vi "FTW-CodeGen-GetTerminals.vi"(0 "Prototype VI":refnum<vi>, 11 "error in":errorcluster) -> (4 "Terms":T5(array[cluster]), 6 "Adaptive Input Terminals":T1[](array[typedef]), 15 "error out":errorcluster)   [LabVIEW 2015]
uses:
  FTW-CodeGen-XNodeAdaptiveTerminal.ctl
  FTW-CodeGen-XNodeAdaptiveTerminal-Controller.ctl
  src/reflection/FTW-Reflection-Types.ctl
  FTW-CodeGen-XNodeAdaptiveTerminal-ControllerBehavior.ctl
  FTW-CodeGen-XNodeAdaptiveTerminal-Dependent.ctl
panel:
  # "Inputs"
  # "Outputs"
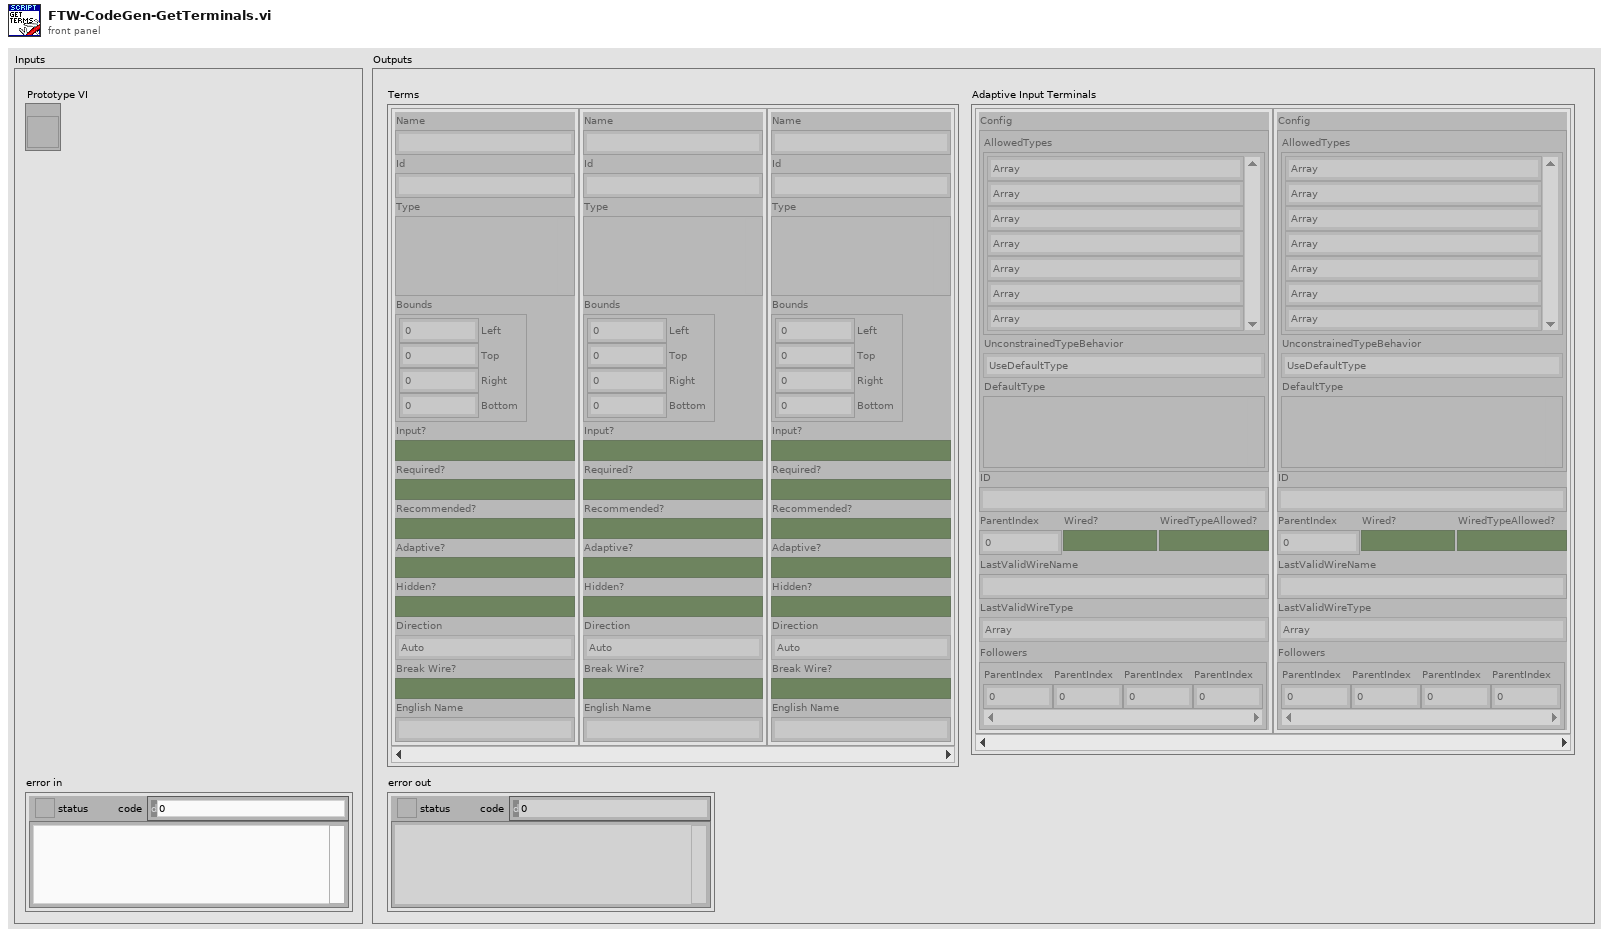
[diagram p1: front panel]
types:
  T1 = typedef "FTW-CodeGen-XNodeAdaptiveTerminal.ctl" = cluster{"Config":T2, "ID":string, "ParentIndex":i32, "Wired?":bool, "WiredTypeAllowed?":bool, "LastValidWireName":string, "LastValidWireType":T3, "Followers":i32[]}
  T2 = typedef "FTW-CodeGen-XNodeAdaptiveTerminal-Controller.ctl" = cluster{"AllowedTypes":T3[], "UnconstrainedTypeBehavior":T4, "DefaultType":variant}
  T3 = typedef "FTW-Reflection-Types.ctl" = enum16{"Unknown", "Void", "Array", "Cluster", "LVObject", "Boolean", "I8", "I16", "I32", "I64", "U8", "U16", "U32", "U64", "SGL", "DBL", "EXT", "CSG", "CDB", "CXT", "FXP", "EnumU8", "EnumU16", "EnumU32", "EnumU64", "SGLwithUnit", "DBLwithUnit", "EXTwithUnit", "CSGwithUnit", "CDBwithUnit", "CXTwithUnit", "String", "Path", "Picture", "Tag", "LVVariant", "Timestamp", "WaveformI8", "WaveformI16", "WaveformI32", "WaveformI64", "WaveformU8", "WaveformU16", "WaveformU32", "WaveformU64", "WaveformSGL", "WaveformDBL", "WaveformEXT", "WaveformCSG", "WaveformCDB", "WaveformCXT", "WaveformDigital", "WaveformUnknownType", "DigitalData", "DynamicData", "ExternalData", "FileByteStream", "TDMStream", "dotNET", "ActiveX", "VIServerReference", "VIReference", "ApplicationInstance", "Menu", "ConnectionDataSocket", "ConnectionVISA", "ConnectionBluetooth", "ConnectionIrDA", "ConnectionTCP", "ConnectionUDP", "ConnectionHTTPClient", "ConnectionFTP", "Occurrence", "Notifier", "Queue", "Rendezvous", "Semaphore", "RTFIFO", "EventPublisher", "EventRegistration", "EventCallback", "DataValueReference", "GenericClass", "GenericClassTag", "GenericClassDeepCopy", "GenericClassFlattened", "GenericClassTagFlattened", "GenericReferenceType", "WindowsRegistry", "OverloadedDatalogRef", "ReferenceUnknownType", "ByteArray", "ConPaneInterface", "FTWObject"}
  T4 = typedef "FTW-CodeGen-XNodeAdaptiveTerminal-ControllerBehavior.ctl" = enum16{"UseDefaultType", "StickyToLastValidType"}
  T5 = cluster{"Name":string, "Id":string, "Type":variant, "Bounds":cluster{"Left":i32, "Top":i32, "Right":i32, "Bottom":i32}, "Input?":bool, "Required?":bool, "Recommended?":bool, "Adaptive?":bool, "Hidden?":bool, "Direction":enum32{"Auto", "Up", "Down", "Left", "Right", "Center"}, "Break Wire?":bool, "English Name":string}[]
  T6 = typedef "FTW-Reflection-ConPaneInterface-Terminal.ctl" = cluster{"Name":string, "LabVIEW Type":T3, "Original Index":i32, "Datatype":variant, "Bounds":cluster{"Left":i32, "Top":i32, "Right":i32, "Bottom":i32}, "Input Stomp Index":i32, "Input":bool, "Wired":bool, "Dynamic Dispatch":bool, "Recommended":bool, "Required":bool, "Stomped":bool, "RSV20":bool, "RSV40":bool}
  T7 = cluster{"Name":string, "Id":string, "Type":variant, "Bounds":cluster{"Left":i32, "Top":i32, "Right":i32, "Bottom":i32}, "Input?":bool, "Required?":bool, "Recommended?":bool, "Adaptive?":bool, "Hidden?":bool, "Direction":enum32{"Auto", "Up", "Down", "Left", "Right", "Center"}, "Break Wire?":bool, "English Name":string}
  T8 = typedef "FTW-CodeGen-XNodeAdaptiveTerminal-Dependent.ctl" = cluster{"FollowingID":string}
  T9 = cluster{"Left":i32, "Top":i32, "Right":i32, "Bottom":i32}
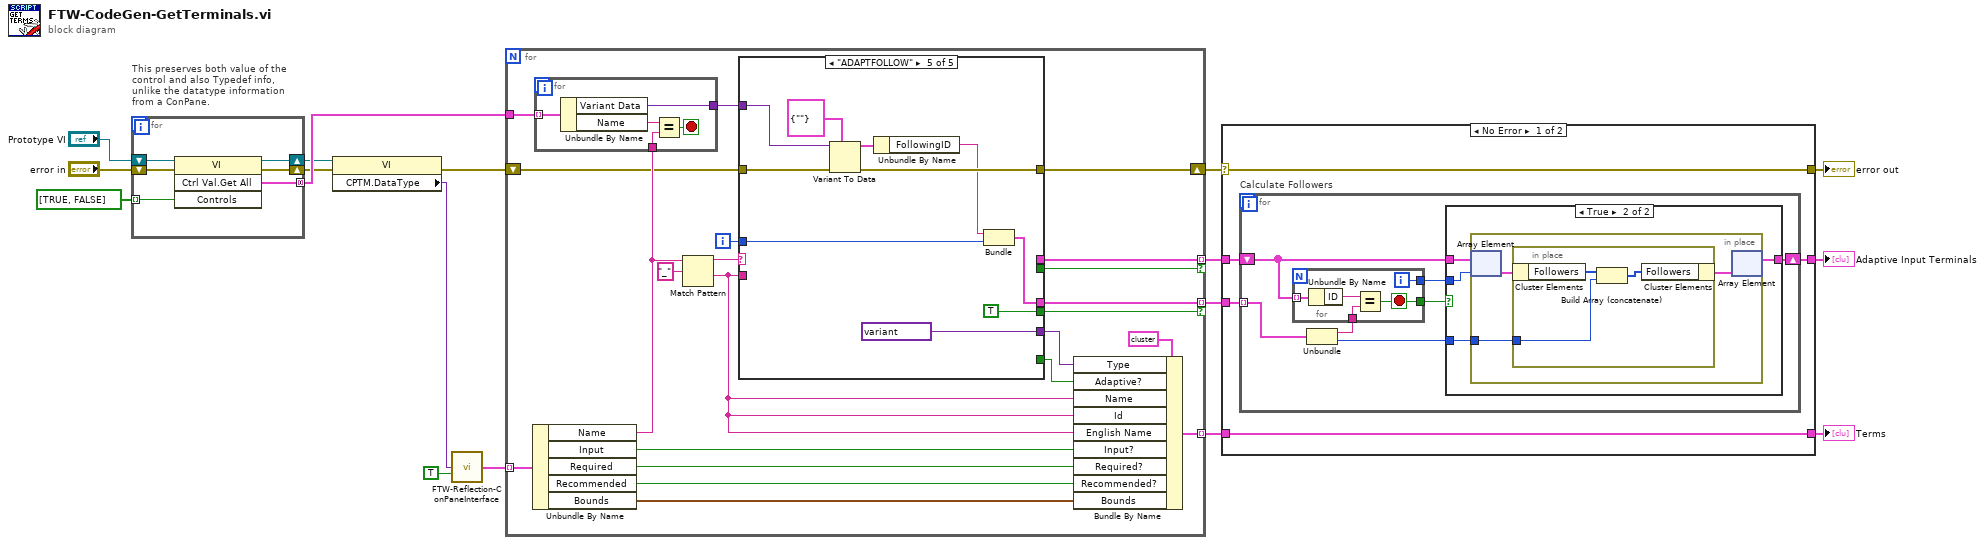
[diagram p0: block diagram]
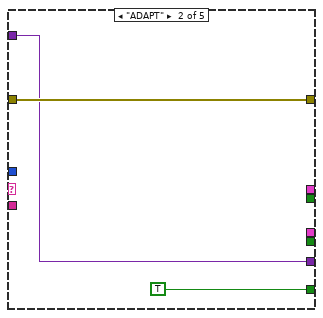
[diagram p3: hidden frame]
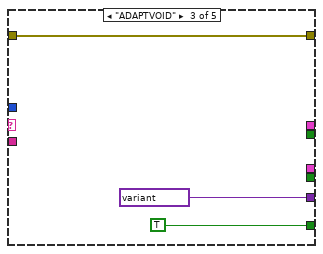
[diagram p4: hidden frame]
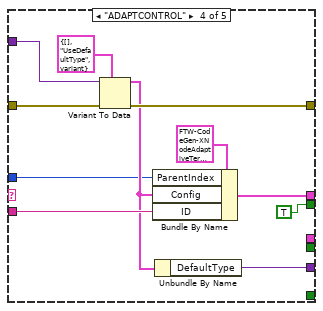
[diagram p5: hidden frame]
diagram:
  n1 = for "This preserves both value of the\ncontrol and also Typedef info,\nunlike the datatype information\nfrom a ConPane." {
    tunnel: [w22] -> w9 mode=concatenating
    tunnel: bool[] [TRUE, FALSE] -> [w19] mode=indexing
    shift-right: [w23] -> w3
    shift-left: "error in" -> [w21]
    shift-right: [w18] -> w4
    shift-left: "Prototype VI" -> [w20]
    n2 = invoke class="VI" method="Ctrl Val.Get All"(reference=w20, error in=w21, "Controls"=w19) -> (reference out=w18:refnum<vi>, error out=w23:errorcluster, "Get All Control Values Variant"=w22:cluster{"Name":string, "Variant Data":variant}[])  [unwired: 1 in, 1 out]
  }
  n3 = property class="VI"(reference=w4, error in=w3) -> (error out=w2:errorcluster, "CPTM.DataType"=w1:variant)  [unwired: 1 out]
  n4 = call "FTW-Reflection-ConPaneInterface.vi"("VI Connector Pane (or VI Reference)"=w1, "Only Return Wired Terminals"=TRUE) -> ("Terminals"=w10:T6[])  [unwired: 11 in, 2 out]
  n5 = for {
    tunnel: [w45] -> w15 mode=indexing
    tunnel: [w44] -> w12 mode=indexing if=w43
    shift-right: [w42] -> w17
    shift-left: w2 -> [w32]
    tunnel: [w41] -> w11 mode=indexing if=w40
    tunnel: w10 -> [w39] mode=indexing
    tunnel: w9 -> [w38]
    i -> [w25]
    n6 = Unbundle By Name(w39) -> ("Name"=w37:string, "Input"=w28:bool, "Required"=w27:bool, "Recommended"=w26:bool, "Bounds"=w24:T9)
    n7 = for {
      tunnel: w37 -> [w49]
      tunnel: w38 -> [w48] mode=indexing
      tunnel: [w46] -> w33
      stop <- w47 stop-if-true
      n8 = Unbundle By Name(w48) -> ("Variant Data"=w46:variant, "Name"=w50:string)
      n9 = Equal?(x=w50, y=w49) -> (x = y?=w47:bool)
    }
    n10 = Match Pattern(string=w37, regular expression="_") -> (before substring=w31:string, after substring=w35:string)  [unwired: 1 in, 2 out]
    n11 = case shown="\"ADAPTFOLLOW\"" w31 {
      tunnel: [_ _ _ w69 _] -> w44
      tunnel: w35 -> [_ _ _ w68 _]
      tunnel: w33 -> [w51 w54 _ w66 w79]
      tunnel: w32 -> [w52 w55 w58 w65 w78]
      tunnel: [w52 w55 w58 w64 w77] -> w42
      tunnel: w25 -> [_ _ _ w59 w74]
      tunnel: [_ _ _ TRUE _] -> w43
      tunnel: [w51 w54 variant w60 variant] -> w30
      tunnel: [_ _ _ _ w72] -> w41
      tunnel: [_ _ _ _ TRUE] -> w40
      tunnel: [_ TRUE TRUE _ _] -> w29
      frame Default {
      }
      frame "ADAPT" {
      }
      frame "ADAPTVOID" {
      }
      frame "ADAPTCONTROL" {
        n12 = Variant To Data(error in=w65, type=T2 {"AllowedTypes"=[], "UnconstrainedTypeBehavior"=enum."UseDefaultType", "DefaultType"=variant(bool FALSE)} ("FTW Adaptive Terminal Config"), Variant=w66) -> (data=w61:T2, error out=w64:errorcluster)
        n13 = Bundle By Name(cluster=T1 {"Config"={"AllowedTypes"=[], "UnconstrainedTypeBehavior"=enum."UseDefaultType", "DefaultType"=variant}, "ID"="", "ParentIndex"=0, "Wired?"=FALSE, "WiredTypeAllowed?"=FALSE, "LastValidWireName"="", "LastValidWireType"=enum."Array", "Followers"=[]}, "ParentIndex"=w59, "Config"=w61, "ID"=w68) -> (w69:T1)
        n14 = Unbundle By Name(w61) -> ("DefaultType"=w60:variant)
      }
      frame "ADAPTFOLLOW" {
        n15 = Variant To Data(error in=w78, type=T8 {"FollowingID"=""} ("FTW Adaptive Terminal Config"), Variant=w79) -> (data=w75:T8, error out=w77:errorcluster)
        n16 = Unbundle By Name(w75) -> ("FollowingID"=w73:string)
        n17 = Bundle("FollowingID"=w73, w74) -> (w72:cluster{"FollowingID":string, i32})  [unwired: 1 in]
      }
    }
    n18 = Bundle By Name(cluster=T7 {"Name"="", "Id"="", "Type"=variant, "Bounds"={"Left"=0, "Top"=0, "Right"=0, "Bottom"=0}, "Input?"=FALSE, "Required?"=FALSE, "Recommended?"=FALSE, "Adaptive?"=FALSE, "Hidden?"=FALSE, "Direction"=enum."Auto", "Break Wire?"=FALSE, "English Name"=""} ("Term 4"), "Type"=w30, "Adaptive?"=w29, "Name"=w35, "Id"=w35, "English Name"=w35, "Input?"=w28, "Required?"=w27, "Recommended?"=w26, "Bounds"=w24) -> (w45:T7)
  }
  n19 = case shown="No Error" w17 {
    selector: w17 -> [w84 w108]
    tunnel: [w84 w108] -> w16
    tunnel: w15 -> [w83 _]
    tunnel: [w83 _] -> w14
    tunnel: [w81 _] -> w13
    tunnel: w12 -> [w82 _]
    tunnel: w11 -> [w80 _]
    frame No Error {
      n20 = for "Calculate Followers" {
        shift-right: [w91] -> w81
        shift-left: w82 -> [w90]
        tunnel: w80 -> [w89] mode=indexing
        n21 = Unbundle(w89) -> ("FollowingID"=w88:string, w85:i32)
        n22 = for {
          tunnel: w88 -> [w106]
          tunnel: w90 -> [w105] mode=indexing
          tunnel: [w104] -> w86
          tunnel: [w103] -> w87
          i -> [w103]
          stop <- w104 stop-if-true
          n23 = Unbundle By Name(w105) -> ("ID"=w107:string)
          n24 = Equal?(x=w107, y=w106) -> (x = y?=w104:bool)
        }
        n25 = case shown="True" w86 {
          tunnel: [w92 w96] -> w91
          tunnel: w90 -> [w92 w95]
          tunnel: w87 -> [_ w94]
          tunnel: w85 -> [_ w93]
          frame False {
          }
          frame True {
            n26 = in-place {
              in-place-border: w93 -> [w98]
              n27 = in-place-array #1(w95, w94) -> (w99:T1)
              n28 = in-place {
                in-place-border: w98 -> [w100]
                n29 = in-place-cluster #2(w99) -> ("Followers"=w102:i32[])
                n30 = Build Array (concatenate)(w102, w100) -> (w101:i32[])
                n31 = in-place-cluster #2("Followers"=w101) -> (w97:T1)
              }
              n32 = in-place-array #1(w97) -> (w96:T1[])  [unwired: 1 out]
            }
          }
        }
      }
    }
    frame Error {
    }
  }
  "error out" <- w16
  "Terms" <- w14
  "Adaptive Input Terminals" <- w13
